vi "5.7-UDP Check Checksum.vi"(0 "CS string in":string) -> (1 "CS string in 2":string, 2 "Boolean":bool)   [LabVIEW 2010]
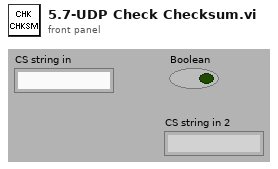
[diagram p1: front panel]
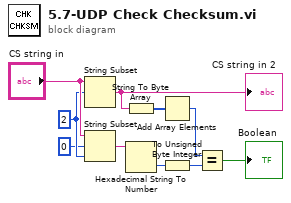
[diagram p0: block diagram]
diagram:
  w3 = 2 ("length (rest)")
  n1 = String Subset(string="CS string in", offset (0)=w3) -> (substring=w4:string)  [unwired: 1 in]
  "CS string in 2" <- w4
  n2 = String Subset(string="CS string in", offset (0)=0, length (rest)=w3) -> (substring=w2:string)
  n3 = String To Byte Array(string=w4) -> (unsigned byte array=w5:u8[])
  n4 = Hexadecimal String To Number(string=w2) -> (number=w7:u32)  [unwired: 2 in, 1 out]
  n5 = Add Array Elements(numeric array=w5) -> (sum=w6:u8)
  n6 = To Unsigned Byte Integer(number=w7) -> (unsigned 8bit integer=w8:u8)
  n7 = Equal?(x=w6, y=w8) -> (x = y?=→"Boolean":bool)
